vi "CreateCore.vi"(7 "Correction Levels":T1, 8 "error in (no error)":errorcluster, 11 "n_qr_codes":u8) -> (0 "error out":errorcluster, 3 "QR Code Encoder":refnum<class "QR Code Encoder.lvclass">)   [LabVIEW 2020, in "feature_detection.lvlib" / "QR Code Encoder.lvclass"]
uses:
  QR Code Encoder.lvclass
  Correction Levels.ctl
  QR Code Encoder.lvclass/QR Code Encoder.ctl
  common/common.lvlib
  common/bin/gartoolkit_fd_32-1.dll
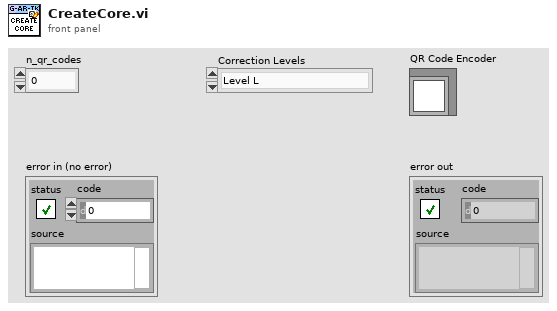
[diagram p1: front panel]
types:
  T1 = typedef "feature_detection.lvlib/QR Code Encoder.lvclass/Correction Levels.ctl" = enum16{"Level L", "Level M", "Level Q", "Level H"}
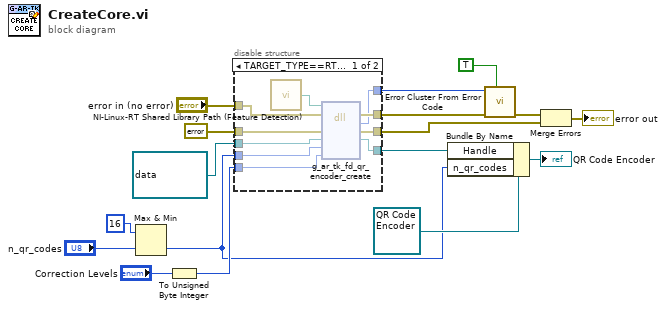
[diagram p0: block diagram]
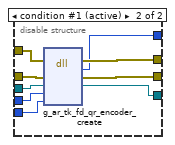
[diagram p2: hidden frame]
diagram:
  n1 = Max & Min(x=u8 16, y="n_qr_codes") -> (min(x,y)=w3:u8)  [unwired: 1 out]
  n2 = To Unsigned Byte Integer(number="Correction Levels") -> (unsigned 8bit integer=w5:u8)
  n3 = disable-structure "Conditional Disable Structure" shown="TARGET_TYPE==RT&&OS==Linux" {
    disable-tunnel: "error in (no error)" -> [w27 w36]
    disable-tunnel: errorcluster {"status"=FALSE, "code"=0, "source"=""} ("error constant") -> [w23 w35]
    disable-tunnel: refnum<data-value> refnum ("EDVR") -> [w22 w34]
    disable-tunnel: [w26 w33] -> w14
    disable-tunnel: [w25 w32] -> w13
    disable-tunnel: [w21 w31] -> w12
    disable-tunnel: [w20 w30] -> w11
    disable-tunnel: w5 -> [w18 w29]
    disable-tunnel: w3 -> [w19 w28]
    frame condition #0 {
      n4 = call "NI-Linux-RT Shared Library Path (Feature Detection).vi"() -> ("Path"=w24:path)
      n5 = dll-call lib="?" fn="g_ar_tk_fd_qr_encoder_create" ("g_ar_toolkit.*.*:g_ar_tk_capture_context_create")(path in=w24, error in=w27, "error_cluster"=w23, "EDVR"=w22, "n_codes"=w19, "error_correction"=w18) -> (error out=w26:errorcluster, w25:i32, "error_cluster"=w20:errorcluster, "EDVR"=w21:refnum<data-value>)  [unwired: 3 in, 1 out]
    }
    frame condition #1 (active) {
      n6 = dll-call lib="C:/serenial/lib/g-augmented-reality-toolkit/LabVIEW/common/bin/gartoolkit_fd_*-1.*" fn="g_ar_tk_fd_qr_encoder_create" ("g_ar_toolkit.*.*:g_ar_tk_capture_context_create")(error in=w36, "error_cluster"=w35, "EDVR"=w34, "n_codes"=w28, "error_correction"=w29) -> (error out=w33:errorcluster, w32:i32, "error_cluster"=w30:errorcluster, "EDVR"=w31:refnum<data-value>)  [unwired: 4 in, 1 out]
    }
  }
  n7 = Bundle By Name(cluster=refnum<class "QR Code Encoder.lvclass"> refnum ("feature_detection.lvlib:QR Code Encoder.lvclass"), "Handle"=w12, "n_qr_codes"=w3) -> (→"QR Code Encoder":refnum<class "QR Code Encoder.lvclass">)
  n8 = call <vilib>:"Error Cluster From Error Code.vi"("show call chain? (False)"=TRUE, "error in (no error)"=w14, "error code (0)"=w13) -> ("error out"=w17:errorcluster)  [unwired: 6 in]
  n9 = Merge Errors(w17, w11) -> (→"error out":errorcluster)
